vi "overlaySwapXY.vi"(1 "overlay in":cluster{"X":i32, "Y":i32, "Z":i32}[](array[cluster])) -> (0 "overlay out":cluster{"X":i32, "Y":i32, "Z":i32}[](array[cluster]))   [LabVIEW 2017]
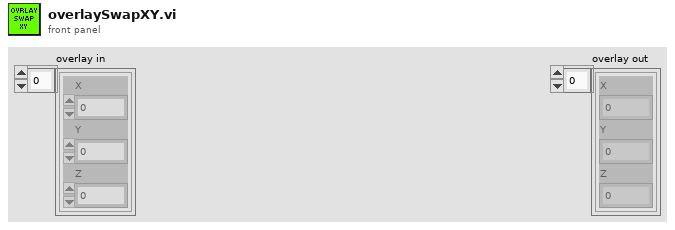
[diagram p1: front panel]
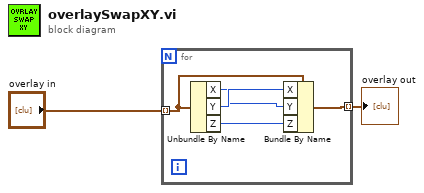
[diagram p0: block diagram]
diagram:
  n1 = for {
    tunnel: "overlay in" -> [w3] mode=indexing
    tunnel: [w5] -> w1 mode=indexing
    n2 = Unbundle By Name(w3) -> ("X"=w6:i32, "Y"=w7:i32, "Z"=w4:i32)
    n3 = Bundle By Name(cluster=w3, "X"=w7, "Y"=w6, "Z"=w4) -> (w5:cluster{"X":i32, "Y":i32, "Z":i32})
  }
  "overlay out" <- w1
